vi "v5.2vi.vi"() -> ()   [LabVIEW 2018]
uses:
  <vilib>/DAQmx/read.llb/DAQmx Read (Analog 1D DBL NChan 1Samp).vi
  <extravilib>/ChannelInstances/High Speed Stream-c(a[.](c(dbl,dbl,dbl,dbl)),stamp,a[.](dbl),c(dbl,dbl,dbl,dbl,dbl,dbl,dbl))/_Read For Replicate.vi
  <extravilib>/ChannelInstances/High Speed Stream-c(a[.](c(dbl,dbl,dbl,dbl)),stamp,a[.](dbl),c(dbl,dbl,dbl,dbl,dbl,dbl,dbl))/Instantiate.vi
  <extravilib>/ChannelInstances/High Speed Stream-c(a[.](c(dbl,dbl,dbl,dbl)),stamp,a[.](dbl),c(dbl,dbl,dbl,dbl,dbl,dbl,dbl))/)Channel.vi
  <extravilib>/ChannelInstances/High Speed Stream-c(a[.](c(dbl,dbl,dbl,dbl)),stamp,a[.](dbl),c(dbl,dbl,dbl,dbl,dbl,dbl,dbl))/Abort Signal/Init Signal.vi
  <vilib>/Utility/file.llb/Write Delimited Spreadsheet (string).vi
  <vilib>/DAQmx/create/channels.llb/DAQmx Create Channel (AI-Temperature-Thermocouple).vi
  <vilib>/DAQmx/configure/timing.llb/DAQmx Timing (Sample Clock).vi
  <vilib>/DAQmx/miscellaneous.llb/DAQmx Fill In Error Info.vi
  <extravilib>/ChannelInstances/High Speed Stream-c(a[.](c(dbl,dbl,dbl,dbl)),stamp,a[.](dbl),c(dbl,dbl,dbl,dbl,dbl,dbl,dbl)).lvlib
  <resource>/objmgr/daqmx.rc
panel:
  out "Line Pressures":T1(graph)
  in  "Boondoggle":dbl(slide) scale=0.0..10.0
  out "Line Temperatures":T1(graph)
  out "Stoichiometric AFR [g/s]":dbl
  in  "stop":bool
  in  "Species List":string[][](table)=[["Custom", "9999999999"], ["Methanol", "6.47"], ["Butanol", "11.2"], ["Diesel", "14.5"], ["Gasoline", "14.7"], ["Propane", "15.67"], ["Methane", "13.19"], ["Hydrogen", "34.3"], ["Ammonia", "6.0466"], ["Pentane", "15.32"], ["Butane", "14.98"], ["Hexane", "15.24"], ["Ethanol", "9"]]
  in  "Tab Control":enum32{"Live Data", "AFR Info", "Setup Lines"}(tab)
  out "Flowrate Data":T2(array[cluster])
  out "AFR Display":T3(array[cluster])
  in  "Line Setup":T4(array[cluster])
  out "Actual Sample Rate":dbl
  out "Export Timestamp":timestamp format="%<%H:%M:%S>T"
  out "Rig Temperatures":T5
  out "UI Timestamp":timestamp format="%<%X\n%x>T"
  out "DAQ Timestamp":timestamp format="%<%H:%M:%S>T"
  in  "file path (dialog if empty)":path
  out "Export Loop Status":T6(ring)
  in  "Start Recording?":bool
  in  "Stop Recording?":bool
  out "Aquisition Loop Status":T7(ring)
  in  "OK Button":bool
  in  "DAQ Properties":cluster{"Sample Rate [Hz]":dbl}={"Sample Rate [Hz]"=1.0} {"Sample Rate [Hz]" min=1.0 max=500.0 step=1.0}
  # "Live \n Live Line Data"
  # "Air-to-Fuel Ratios for each Line"
  # "Line Setup"
  # "Rig Temperatures [ °C]"
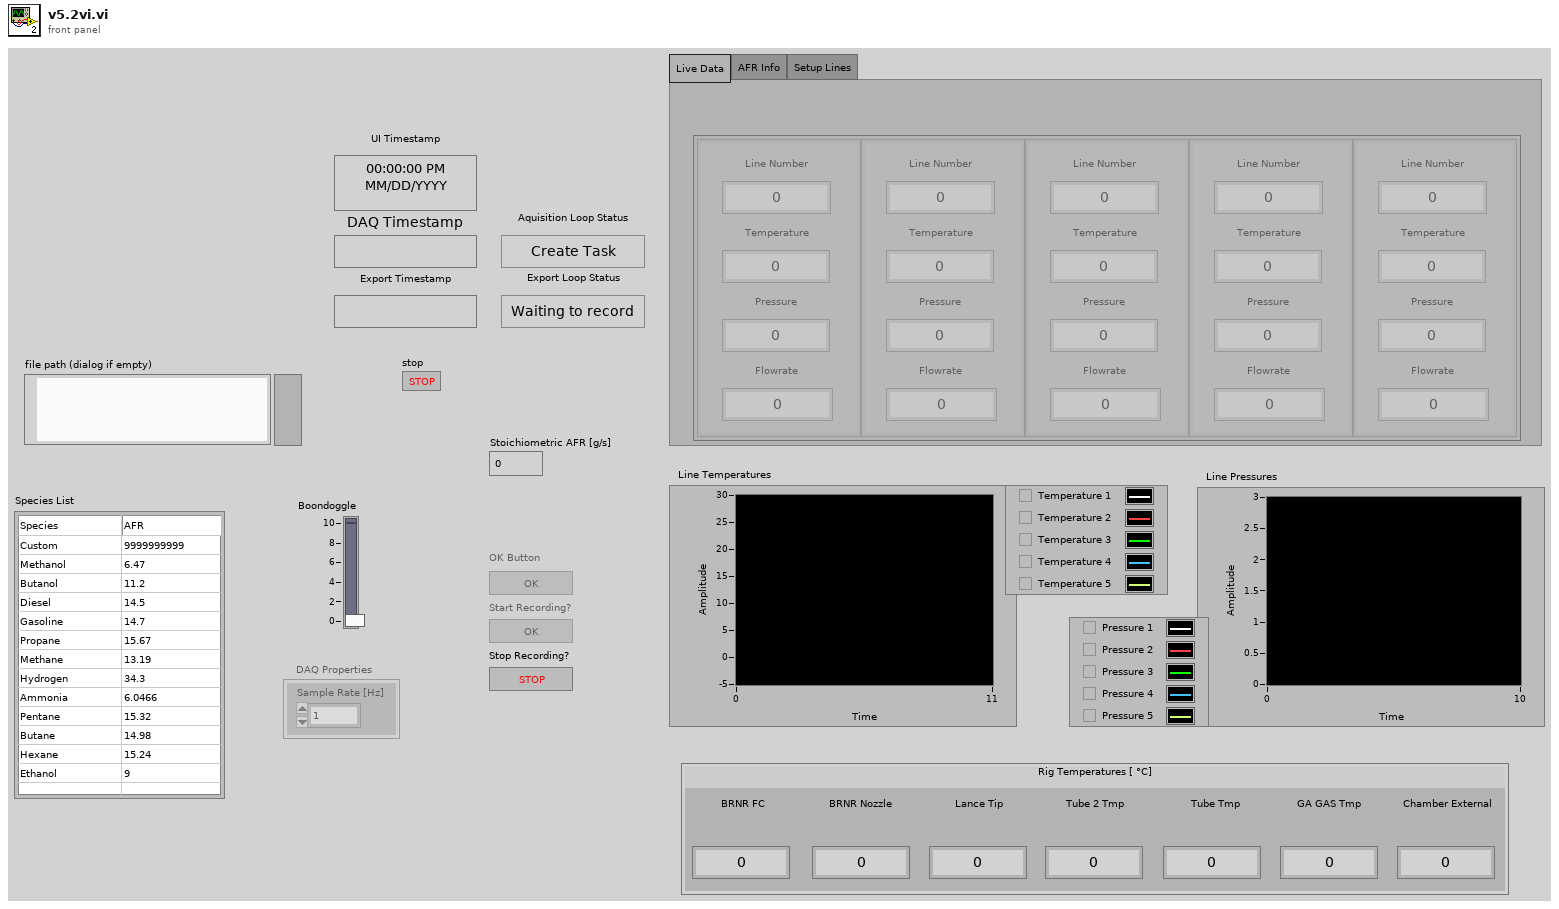
[diagram p1: front panel]
types:
  T1 = cluster{"[0]":dbl, "[1]":dbl, "[2]":dbl, "[3]":dbl, "[4]":dbl, "[5]":dbl, "[6]":dbl, "[7]":dbl, "[8]":dbl}
  T2 = cluster{"Line Number":dbl, "Temperature":dbl, "Pressure":dbl, "Flowrate":dbl}[]
  T3 = cluster{"Line Number":i32, "AFR":dbl, "Species":enum16{"Empty (Not used)", "Custom", "Methanol", "Ethanol", "Butanol", "Diesel", "Gasoline", "Propane", "Methane", "Hydrogen", "Pentane", "Butane", "Hexane"}}[]
  T4 = cluster{"Custom AFR":dbl, "Species":enum16{"Empty (Not used)", "Custom", "Methanol", "Ethanol", "Butanol", "Diesel", "Gasoline", "Propane", "Methane", "Hydrogen", "Pentane", "Butane", "Hexane"}}[]
  T5 = cluster{"BRNR FC":dbl, "BRNR Nozzle":dbl, "Lance Tip":dbl, "Tube 2 Tmp":dbl, "Tube Tmp":dbl, "GA GAS Tmp":dbl, "Chamber External":dbl}
  T6 = enum16{"Waiting to record", "Creating Spreadsheet", "Recording", "Finished Recording"}
  T7 = enum16{"Create Task", "Change Settings", "Check Settings", "Read Data", "End Task"}
  T8 = enum8{"Enabled", "Disabled", "Disabled and Grayed Out"}
  T9 = cluster{"Line":i32, "AFR":dbl, "Species":enum16{"Empty (Not used)", "Custom", "Methanol", "Ethanol", "Butanol", "Diesel", "Gasoline", "Propane", "Methane", "Hydrogen", "Pentane", "Butane", "Hexane"}}
  T10 = enum16{"Empty (Not used)", "Custom", "Methanol", "Ethanol", "Butanol", "Diesel", "Gasoline", "Propane", "Methane", "Hydrogen", "Pentane", "Butane", "Hexane"}
  T11 = cluster{"Flowrate Data":cluster{"Line Number":dbl, "Temperature":dbl, "Pressure":dbl, "Flowrate":dbl}[], "Current Time":timestamp, "DAQmx Data":dbl[], "Rig Temperatures":cluster{"BRNR FC":dbl, "BRNR Nozzle":dbl, "Lance Tip":dbl, "Tube 2 Tmp":dbl, "Tube Tmp":dbl, "GA GAS Tmp":dbl, "Chamber External Temp":dbl}}
  T12 = cluster{"BRNR FC":dbl, "BRNR Nozzle":dbl, "Lance Tip":dbl, "Tube 2 Tmp":dbl, "Tube Tmp":dbl, "GA GAS Tmp":dbl, "Chamber External Temp":dbl}
  T13 = typedef "High Speed Stream-c(a[.](c(dbl,dbl,dbl,dbl)),stamp,a[.](dbl),c(dbl,dbl,dbl,dbl,dbl,dbl,dbl)).lvlib/)Channel.ctl" = refnum<queue>
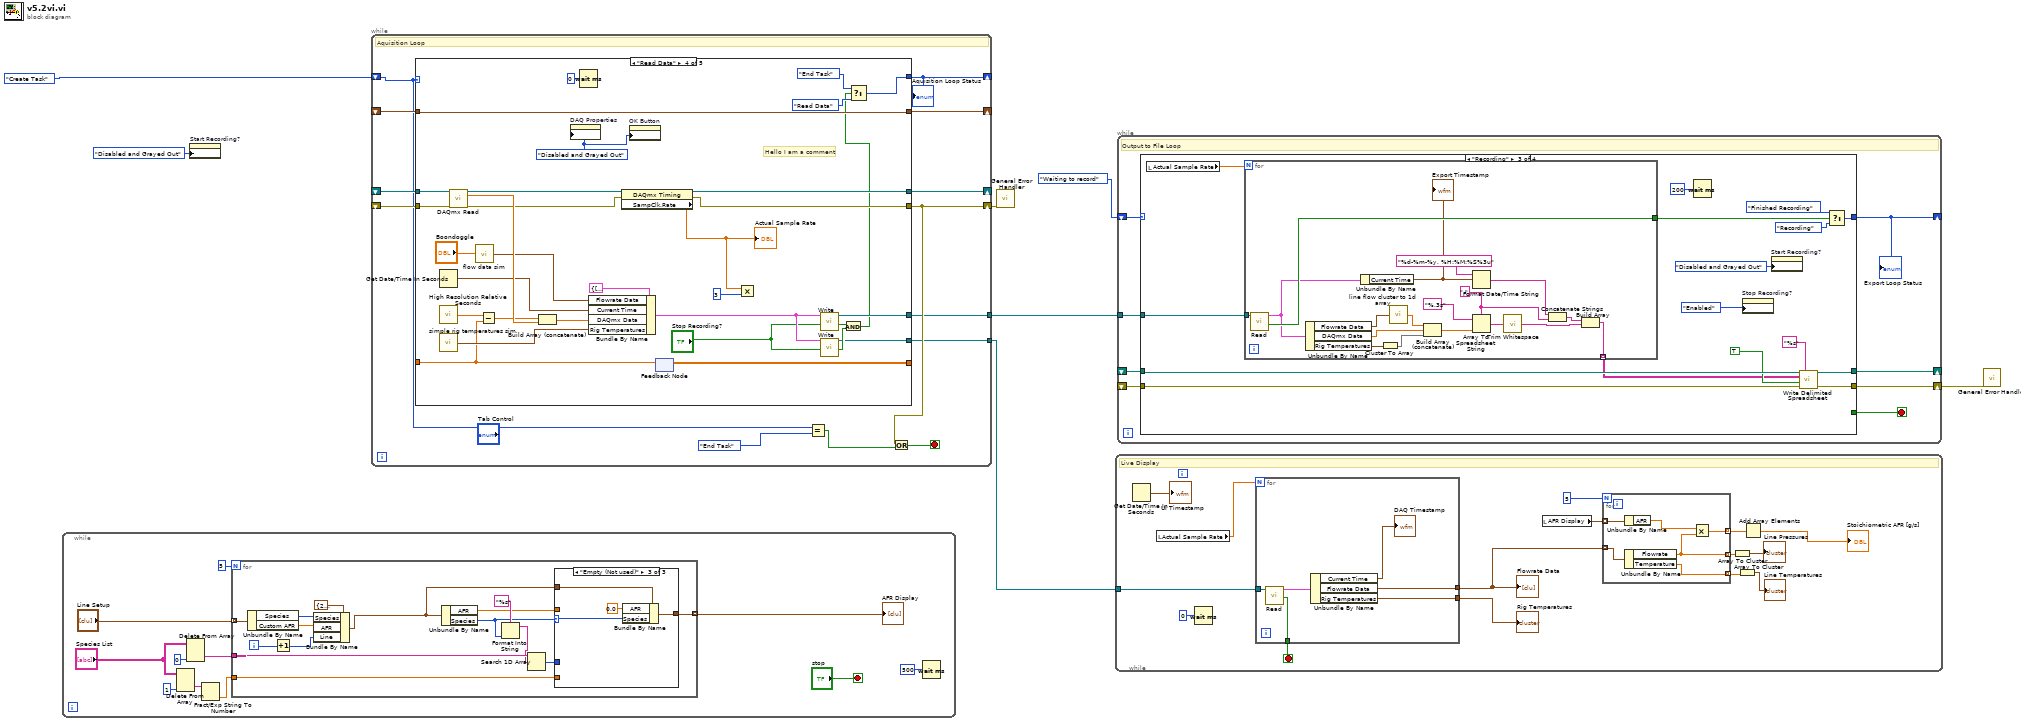
[diagram p0: block diagram]
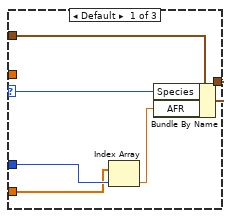
[diagram p2: hidden frame]
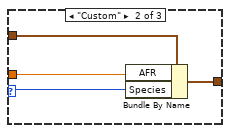
[diagram p3: hidden frame]
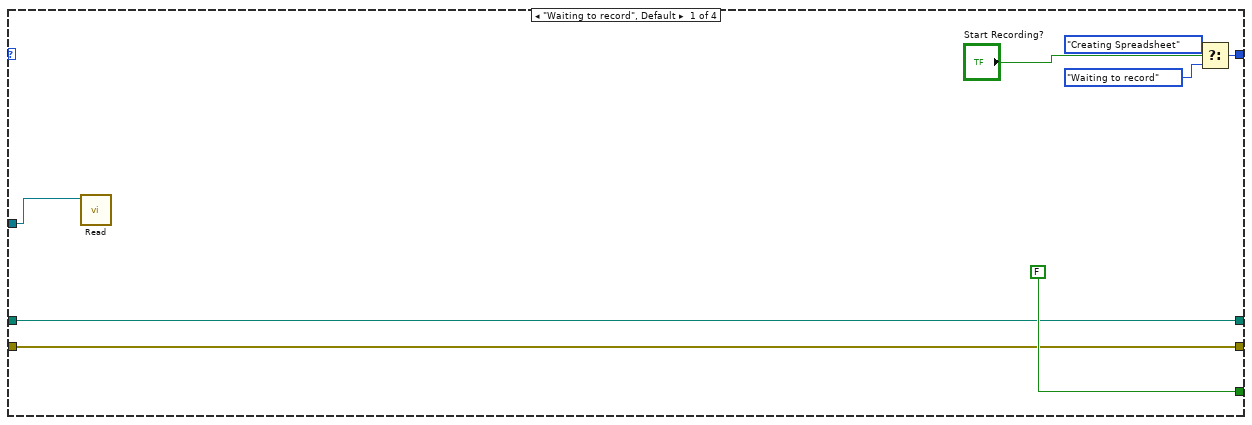
[diagram p4: hidden frame]
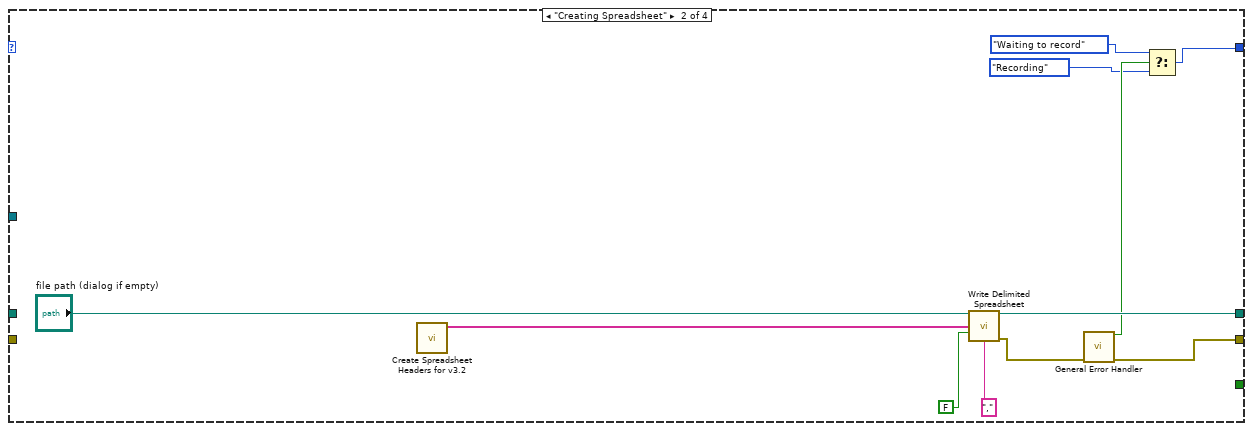
[diagram p5: hidden frame]
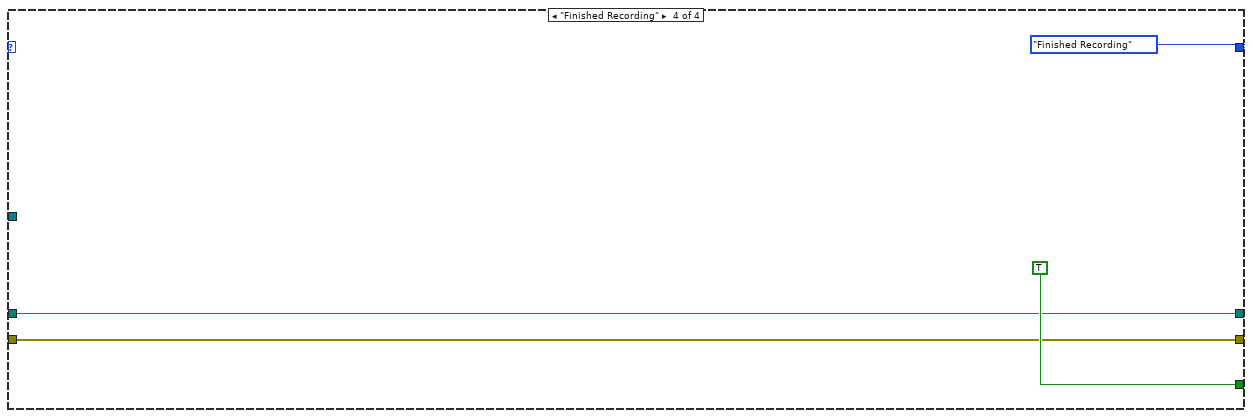
[diagram p6: hidden frame]
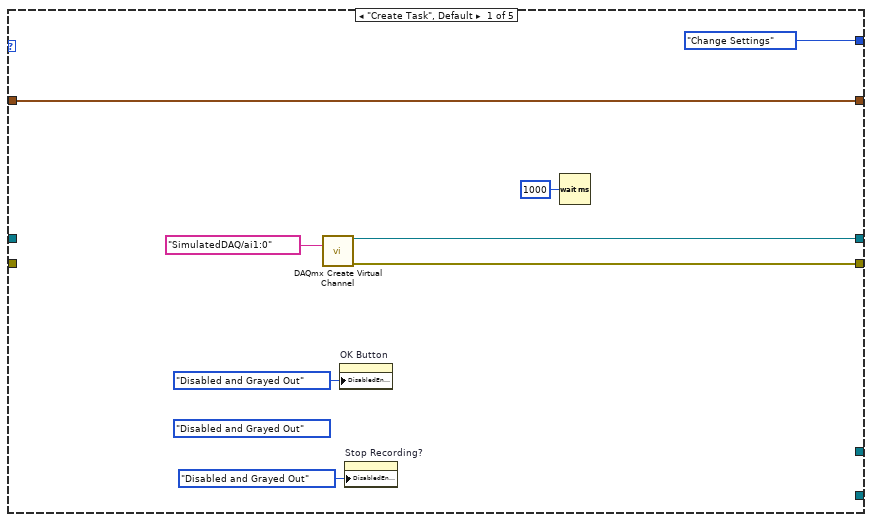
[diagram p7: hidden frame]
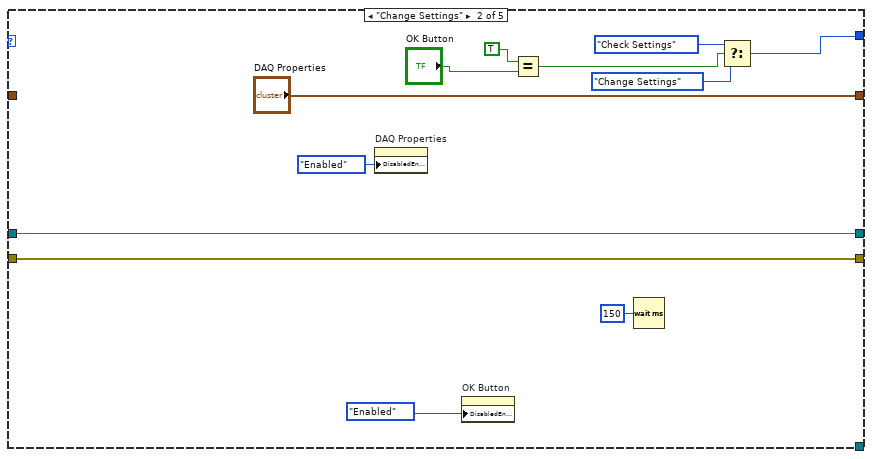
[diagram p8: hidden frame]
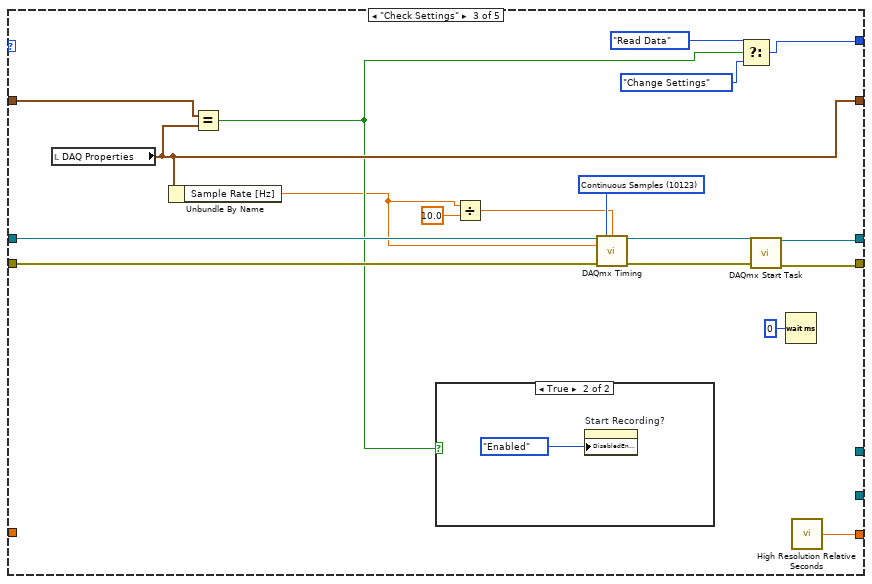
[diagram p9: hidden frame]
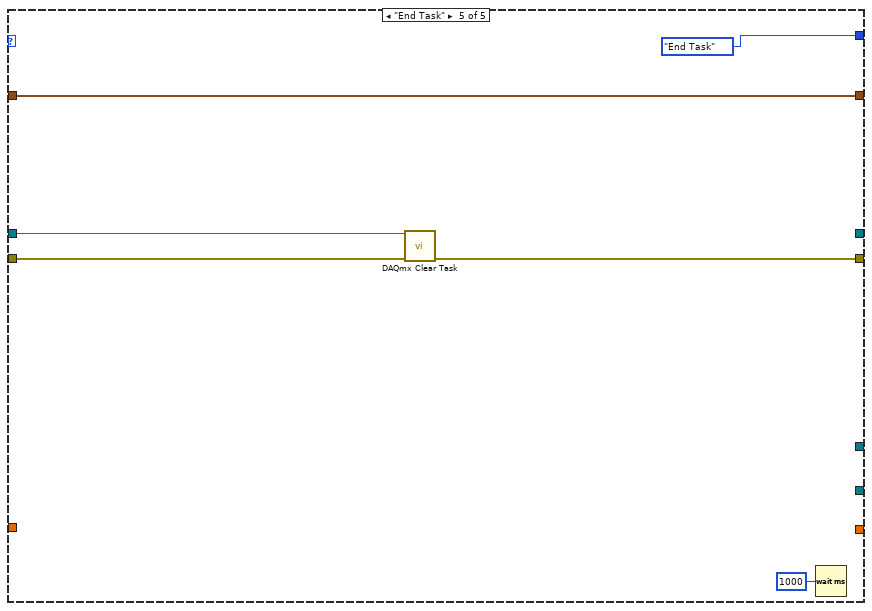
[diagram p11: hidden frame]
diagram:
  n1 = while {
    stop <- "stop" stop-if-true
    n2 = Delete From Array(array="Species List", index (col)=1 ("disabled index (col)")) -> (deleted portion=w13:string[])  [unwired: 2 in, 1 out]
    n3 = Delete From Array(array="Species List", index (col)=0) -> (deleted portion=w14:string[])  [unwired: 2 in, 1 out]
    n4 = Fract/Exp String To Number(string=w13) -> (number=w12:dbl[])  [unwired: 3 in, 1 out]
    n5 = for {
      N: 5 -> [_]
      tunnel: w14 -> [w32]
      tunnel: w12 -> [w29]
      tunnel: "Line Setup" -> [w22] mode=indexing
      tunnel: [w19] -> w8 mode=indexing
      i -> [w21]
      n6 = Unbundle By Name(w22) -> ("Species"=w26:T10, "Custom AFR"=w25:dbl)
      n7 = Increment(x=w21) -> (x+1=w23:i32)
      n8 = Bundle By Name(cluster=T9 {"Line"=2, "AFR"=1.0, "Species"=enum."Pentane"} ("AFR Inputs"), "Species"=w26, "AFR"=w25, "Line"=w23) -> (w20:T9)
      n9 = Unbundle By Name(w20) -> ("AFR"=w30:dbl, "Species"=w27:T10)
      n10 = Format Into String(format string="%s", w27) -> (resulting string=w31:string)  [unwired: 2 in, 1 out]
      n11 = Search 1D Array(1D array=w32, element=w31) -> (index of element=w28:i32)  [unwired: 1 in]
      n12 = case shown="\"Empty (Not used)\"" w27 {
        selector: w27 -> [w36 w40 w45]
        tunnel: w30 -> [_ w43 _]
        tunnel: w29 -> [w38 _ _]
        tunnel: w28 -> [w39 _ _]
        tunnel: [w34 w42 w47] -> w19
        tunnel: w20 -> [w35 w41 w46]
        frame Default {
          n13 = Index Array(array=w38, index=w39) -> (element=w37:dbl)
          n14 = Bundle By Name(cluster=w35, "Species"=w36, "AFR"=w37) -> (w34:T9)
        }
        frame "Custom" {
          n15 = Bundle By Name(cluster=w41, "AFR"=w43, "Species"=w40) -> (w42:T9)
        }
        frame "Empty (Not used)" {
          n16 = Bundle By Name(cluster=w46, "AFR"=0.0, "Species"=w45) -> (w47:T9)
        }
      }
    }
    "AFR Display" <- w8
    n17 = Wait (ms)(milliseconds to wait=u32 500) -> ()  [unwired: 1 out]
  }
  n18 = property on="Start Recording?" class="Bool"("DisabledEnum"=T8."Disabled and Grayed Out" ("Disabled")) -> ()  [unwired: 2 in, 2 out]
  n19 = while {
    shift-right: [w57] -> _
    shift-left: T7."Create Task" -> [w53]
    shift-right: [w62] -> _
    shift-left: _ -> [w60]
    shift-right: [w56] -> w3
    shift-left: _ -> [w59]
    shift-right: [w61] -> _
    shift-left: _ -> [w58]
    tunnel: [w52] -> w5
    tunnel: [w51] -> w1
    stop <- w48 stop-if-true
    # "Aquisition Loop"
    n20 = feedback #1() -> (w49:dbl)  [unwired: 1 in]
    n21 = case shown="\"Read Data\"" w53 {
      tunnel: [w70 w82 w90 w113 _] -> w62
      tunnel: [w69 w81 w89 w114 w138] -> w56
      tunnel: [T7."Change Settings" w75 w96 w128 T7."End Task"] -> w57
      tunnel: [w66 "DAQ Properties" w93 w130 w137] -> w61
      tunnel: w60 -> [_ w82 w95 w132 w135]
      tunnel: w59 -> [_ w81 w94 w131 w134]
      tunnel: w58 -> [w66 _ w100 w130 w137]
      tunnel: [_ _ _ w120 _] -> w52
      tunnel: [_ _ _ w111 _] -> w51
      tunnel: [_ _ w83 w106 _] -> w50
      tunnel: w49 -> [_ _ _ w106 _]
      frame "Create Task", Default {
        (unwired) T8."Disabled and Grayed Out" ("Disabled")
        n22 = call-poly <vilib>:"DAQmx Create Virtual Channel.vi"("physical channels"=tag "SimulatedDAQ/ai1:0") -> ("task out"=w70:refnum<k21>, "error out"=w69:errorcluster)  [unwired: 13 in]
        n23 = property on="OK Button" class="Bool"("DisabledEnum"=T8."Disabled and Grayed Out" ("Disabled")) -> ()  [unwired: 2 in, 2 out]
        n24 = property on="Stop Recording?" class="Bool"("DisabledEnum"=T8."Disabled and Grayed Out" ("Disabled")) -> ()  [unwired: 2 in, 2 out]
        n25 = Wait (ms)(milliseconds to wait=u32 1000) -> ()  [unwired: 1 out]
      }
      frame "Change Settings" {
        n26 = property on="DAQ Properties" class="Clust (strict)"("DisabledEnum"=T8."Enabled" ("Disabled")) -> ()  [unwired: 2 in, 2 out]
        n27 = property on="OK Button" class="Bool"("DisabledEnum"=T8."Enabled" ("Disabled")) -> ()  [unwired: 2 in, 2 out]
        n28 = Equal?(x=TRUE, y="OK Button") -> (x = y?=w77:bool)
        n29 = Wait (ms)(milliseconds to wait=u32 150) -> ()  [unwired: 1 out]
        n30 = Select(t=T7."Check Settings", s=w77, f=T7."Change Settings") -> (s? t:f=w75:T7)
      }
      frame "Check Settings" {
        w88 = 10123 items=["Finite Samples"=10178, "Continuous Samples"=10123, "Hardware Timed Single Point"=12522] ("sample mode")
        n31 = local read "DAQ Properties"() -> (w93:cluster{"Sample Rate [Hz]":dbl})
        n32 = Unbundle By Name(w93) -> ("Sample Rate [Hz]"=w85:dbl)
        n33 = Equal?(x=w100, y=w93) -> (x = y?=w87:bool)
        n34 = case shown="True" w87 {
          frame False {
          }
          frame True {
            n35 = property on="Start Recording?" class="Bool"("DisabledEnum"=T8."Enabled" ("Disabled")) -> ()  [unwired: 2 in, 2 out]
          }
        }
        n36 = Divide(x=w85, y=10.0) -> (x/y=w84:dbl)
        n37 = call-poly <vilib>:"DAQmx Timing.vi"("task/channels in"=w95, "sample mode"=w88, "samples per channel"=w84, "rate"=w85, "error in"=w94) -> ("task out"=w92:refnum<k21>, "error out"=w91:errorcluster)  [unwired: 9 in]
        n38 = Select(t=T7."Read Data", s=w87, f=T7."Change Settings") -> (s? t:f=w96:T7)
        n39 = call <vilib>:"DAQmx Start Task.vi"("task/channels in"=w92, "error in"=w91) -> ("task out"=w90:refnum<k21>, "error out"=w89:errorcluster)  [unwired: 12 in]
        n40 = Wait (ms)(milliseconds to wait=u32 0) -> ()  [unwired: 1 out]
        n41 = call <vilib>:"High Resolution Relative Seconds.vi"() -> ("relative seconds"=w83:dbl)
      }
      frame "Read Data" {
        w119 = T8."Disabled and Grayed Out" ("Disabled")
        # "Hello I am a comment"
        n42 = Get Date/Time In Seconds() -> (seconds since 1Jan1904=w123:timestamp)
        n43 = call <vilib>:"High Resolution Relative Seconds.vi"() -> ("relative seconds"=w110:dbl)
        n44 = call "simple rig temperatures sim.vi"() -> ("Rig Temperatures"=w121:T12)
        n45 = call-poly <vilib>:"DAQmx Read.vi"("task/channels in"=w132, "error in"=w131) -> ("task out"=w115:refnum<k21>, "data"=w125:dbl[], "error out"=w112:errorcluster)  [unwired: 11 in]
        n46 = call "flow data sim.vi"("Boondoggle Input"="Boondoggle") -> ("Flowrate Data"=w122:T2)
        n47 = Subtract(x=w110, y=w106) -> (x-y=w107:dbl)
        n48 = Build Array (concatenate)(w107, w125) -> (w108:dbl[])
        n49 = property on="DAQ Properties" class="Clust (strict)"("DisabledEnum"=w119) -> ()  [unwired: 2 in, 2 out]
        n50 = Wait (ms)(milliseconds to wait=u32 0) -> ()  [unwired: 1 out]
        n51 = Bundle By Name(cluster=T11 {"Flowrate Data"=[{"Line Number"=1.0, "Temperature"=17.480721541683437, "Pressure"=24.0, "Flowrate"=0.0}, {"Line Number"=2.0, "Temperature"=21.850901927104296, "Pressure"=30.0, "Flowrate"=0.0}, {"Line Number"=3.0, "Temperature"=26.221082312525155, "Pressure"=36.0, "Flowrate"=0.0}, {"Line Number"=4.0, "Temperature"=30.591262697946018, "Pressure"=42.00000000000001, "Flowrate"=0.0}, {"Line Number"=5.0, "Temperature"=34.96144308336687, "Pressure"=48.0, "Flowrate"=0.0}], "Current Time"=timestamp(0 s since 1904-01-01), "DAQmx Data"=[], "Rig Temperatures"={"BRNR FC"=0.0, "BRNR Nozzle"=0.0, "Lance Tip"=0.0, "Tube 2 Tmp"=0.0, "Tube Tmp"=0.0, "GA GAS Tmp"=0.0, "Chamber External Temp"=0.0}}, "Flowrate Data"=w122, "Current Time"=w123, "DAQmx Data"=w108, "Rig Temperatures"=w121) -> (w118:T11)
        n52 = property class="DAQmx Timing"(reference=w115, error in=w112) -> (reference out=w113:refnum<k21>, error out=w114:errorcluster, "SampClk.Rate"=w105:dbl)
        "Actual Sample Rate" <- w105
        n53 = property on="OK Button" class="Bool"("DisabledEnum"=w119) -> ()  [unwired: 2 in, 2 out]
        n54 = Multiply(x=w105, y=3) -> ()  [unwired: 1 out]
        n55 = call <extravilib>:"Write.vi"("last element? (F)"="Stop Recording?", "element"=w118) -> ("done?"=w117:bool, "channel"=w120:T13)  [unwired: 7 in, 1 out]
        n56 = call <extravilib>:"Write.vi"("last element? (F)"="Stop Recording?", "element"=w118) -> ("done?"=w116:bool, "channel"=w111:T13)  [unwired: 7 in, 1 out]
        n57 = And(x=w117, y=w116) -> (x .and. y?=w109:bool)
        n58 = Select(t=T7."End Task", s=w109, f=T7."Read Data") -> (s? t:f=w128:T7)
      }
      frame "End Task" {
        n59 = call <vilib>:"DAQmx Clear Task.vi"("task in"=w135, "error in"=w134) -> ("error out"=w138:errorcluster)  [unwired: 13 in]
        n60 = Wait (ms)(milliseconds to wait=u32 1000) -> ()  [unwired: 1 out]
      }
    }
    "Aquisition Loop Status" <- w57
    n61 = feedback-in #1(w50) -> ()
    n62 = Equal?(x=w53, y=T7."End Task") -> (x = y?=w54:bool)
    n63 = Or(x=w56, y=w54) -> (x .or. y?=w48:bool)
  }
  n64 = call <vilib>:"General Error Handler.vi"("error in (no error)"=w3) -> ()  [unwired: 10 in, 5 out]
  n65 = while {
    tunnel: w1 -> [w150]
    stop <- w153 stop-if-true
    # "Live Display"
    n66 = Get Date/Time In Seconds() -> (seconds since 1Jan1904=→"UI Timestamp":timestamp)
    n67 = local read "Actual Sample Rate"() -> (w149:dbl)
    n68 = Wait (ms)(milliseconds to wait=u32 0) -> ()  [unwired: 1 out]
    n69 = for {
      N: w149 -> [_]
      tunnel: [w165] -> w153
      tunnel: w150 -> [w163]
      tunnel: [w160] -> w143
      tunnel: [w162] -> w148
      n70 = call <extravilib>:"Read.vi"("channel"=w163) -> ("done?"=w165:bool, "element"=w164:T11)  [unwired: 6 in, 3 out]
      n71 = Unbundle By Name(w164) -> ("Current Time"=→"DAQ Timestamp":timestamp, "Flowrate Data"=w160:T2, "Rig Temperatures"=w162:T12)
    }
    "Flowrate Data" <- w143
    "Rig Temperatures" <- w148
    n72 = local read "AFR Display"() -> (w146:T3)
    n73 = for {
      N: 5 -> [_]
      tunnel: w146 -> [w159] mode=indexing
      tunnel: w143 -> [w158] mode=indexing
      tunnel: [w156] -> w145 mode=indexing
      tunnel: [w155] -> w141 mode=indexing
      tunnel: [w154] -> w142 mode=indexing
      n74 = Unbundle By Name(w159) -> ("AFR"=w157:dbl)
      n75 = Unbundle By Name(w158) -> ("Flowrate"=w154:dbl, "Temperature"=w155:dbl)
      n76 = Multiply(x=w157, y=w154) -> (x*y=w156:dbl)
    }
    n77 = Array To Cluster(array=w142) -> (cluster=→"Line Pressures":T1)
    n78 = Array To Cluster(array=w141) -> (cluster=→"Line Temperatures":T1)
    n79 = Add Array Elements(numeric array=w145) -> (sum=→"Stoichiometric AFR [g/s]":dbl)
  }
  n80 = while {
    shift-right: [w173] -> _
    shift-left: T6."Waiting to record" -> [w172]
    tunnel: w5 -> [w170]
    shift-right: [w168] -> _
    shift-left: _ -> [w169]
    shift-right: [w167] -> w4
    shift-left: _ -> [w166]
    stop <- w171 stop-if-true
    # "Output to File Loop"
    n81 = case shown="\"Recording\"" w172 {
      tunnel: [w178 w184 w207 T6."Finished Recording"] -> w173
      tunnel: [FALSE _ _ TRUE] -> w171
      tunnel: w170 -> [w174 _ w204 _]
      tunnel: w169 -> [w176 _ w201 w228]
      tunnel: [w176 w192 w202 w228] -> w168
      tunnel: [w175 w186 w197 w227] -> w167
      tunnel: w166 -> [w175 _ w200 w227]
      frame "Waiting to record", Default {
        n82 = call <extravilib>:"Read.vi"("channel"=w174) -> ()  [unwired: 6 in, 5 out]
        n83 = Select(t=T6."Creating Spreadsheet", s="Start Recording?", f=T6."Waiting to record") -> (s? t:f=w178:T6)
      }
      frame "Creating Spreadsheet" {
        n84 = call "Create Spreadsheet Headers for v3.2.vi"() -> ("Array"=w191:string[])  [unwired: 11 in]
        n85 = call-poly <vilib>:"Write Delimited Spreadsheet.vi"("file path (dialog if empty)"="file path (dialog if empty)", "1D data"=w191, "append to file? (new file:F)"=FALSE, "delimiter (\\t)"="," ("delimiter (\\t)")) -> ("new file path (Not A Path if cancelled)"=w192:path, "error out"=w187:errorcluster)  [unwired: 10 in]
        n86 = call <vilib>:"General Error Handler.vi"("error in (no error)"=w187) -> ("error?"=w185:bool, "error out"=w186:errorcluster)  [unwired: 10 in, 3 out]
        n87 = Select(t=T6."Waiting to record", s=w185, f=T6."Recording") -> (s? t:f=w184:T6)
      }
      frame "Recording" {
        n88 = local read "Actual Sample Rate"() -> (w194:dbl)
        n89 = for {
          N: w194 -> [_]
          tunnel: w204 -> [w225]
          tunnel: [w224] -> w203
          tunnel: [w209] -> w195 mode=indexing
          w214 = "," ("delimiter (Tab)")
          n90 = call <extravilib>:"Read.vi"("channel"=w225) -> ("done?"=w224:bool, "element"=w222:T11)  [unwired: 6 in, 3 out]
          n91 = Unbundle By Name(w222) -> ("Flowrate Data"=w223:T2, "DAQmx Data"=w220:dbl[], "Rig Temperatures"=w226:T12)
          n92 = Unbundle By Name(w222) -> ("Current Time"=w215:timestamp)
          "Export Timestamp" <- w215
          n93 = Cluster To Array(cluster=w226) -> (array=w221:dbl[])
          n94 = call "line flow cluster to 1d array.vi"("Flowrate Data"=w223) -> ("Array"=w219:dbl[])
          n95 = Build Array (concatenate)(w219, w220, w221) -> (w212:dbl[])
          n96 = Format Date/Time String(time format string (%c)="%d-%m-%y, %H:%M:%S%3u", seconds (now)=w215) -> (date/time string=w213:string)  [unwired: 1 in]
          n97 = Array To Spreadsheet String(delimiter (Tab)=w214, array=w212, 3:"%.3s" ("format string")) -> (spreadsheet string=w218:string)
          n98 = call <vilib>:"Trim Whitespace.vi"("string"=w218) -> ("trimmed string"=w210:string)  [unwired: 1 in]
          n99 = Concatenate Strings(w213, w214) -> (w211:string)
          n100 = Build Array(w211, w210) -> (w209:string[])
        }
        n101 = Wait (ms)(milliseconds to wait=u32 200) -> ()  [unwired: 1 out]
        n102 = property on="Stop Recording?" class="Bool"("DisabledEnum"=T8."Enabled" ("Disabled")) -> ()  [unwired: 2 in, 2 out]
        n103 = property on="Start Recording?" class="Bool"("DisabledEnum"=T8."Disabled and Grayed Out" ("Disabled")) -> ()  [unwired: 2 in, 2 out]
        n104 = call-poly <vilib>:"Write Delimited Spreadsheet.vi"("file path (dialog if empty)"=w201, "format (%s)"="%s", "2D data"=w195, "append to file? (new file:F)"=TRUE, "error in (no error)"=w200) -> ("new file path (Not A Path if cancelled)"=w202:path, "error out"=w197:errorcluster)  [unwired: 9 in]
        n105 = Select(t=T6."Finished Recording", s=w203, f=T6."Recording") -> (s? t:f=w207:T6)
      }
      frame "Finished Recording" {
      }
    }
    "Export Loop Status" <- w173
  }
  n106 = call <vilib>:"General Error Handler.vi"("error in (no error)"=w4) -> ()  [unwired: 10 in, 5 out]
